vi "Add IP Address.vi"(7 "Connected(F)":bool, 8 "error in":errorcluster, 10 "Alias":string, 11 "IP Address":string) -> (0 "error out":errorcluster, 2 "Alias to Add":string, 3 "IP to Add":string)   [LabVIEW 2014, in "Raspberry Pi Compatible Compiler for LabVIEW.lvlib"]
uses:
  Raspberry Pi Compatible Compiler for LabVIEW.lvlib
  RasPi_Services/Autodetect/Autodetect.lvlib
panel:
  out "Animated Image":i16(ring) caption="Ring 2"
  in  "Cancel":bool
  in  "Add Ip":bool
  in  "Veirfy Connectivity":bool
  in  "Alias":string
  in  "IP Address":string
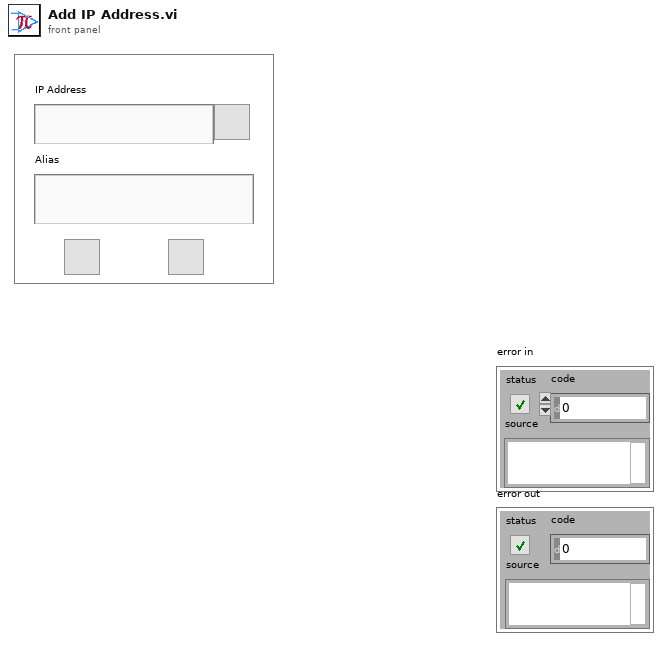
[diagram p1: front panel]
types:
  T1 = enum8{"Enabled", "Disabled", "Disabled and Grayed Out"}
  T2 = typedef "Raspberry Pi Compatible Compiler for LabVIEW.lvlib/Autodetect.lvlib/UDP_Response_TD.ctl" = cluster{"IP address":string, "Port":u16, "response":string}
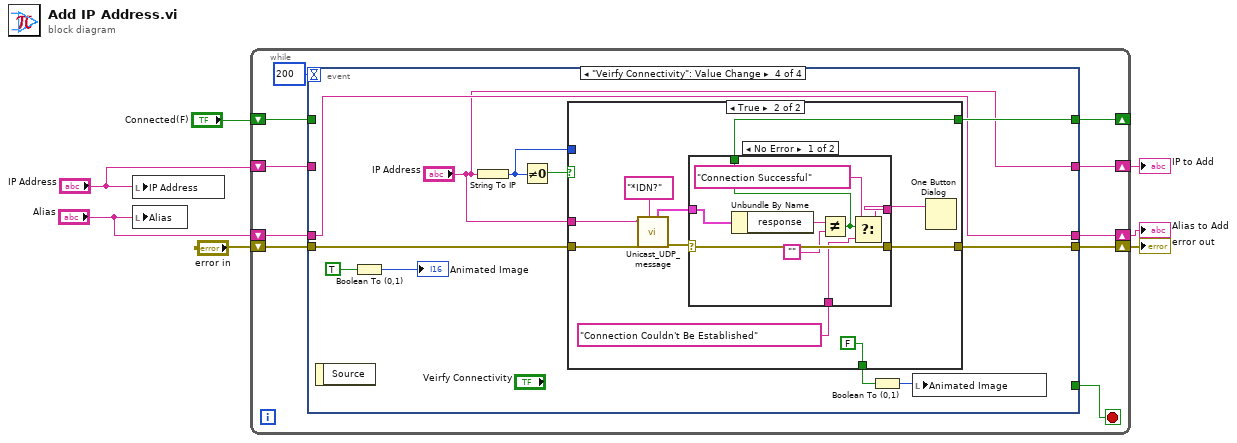
[diagram p0: block diagram]
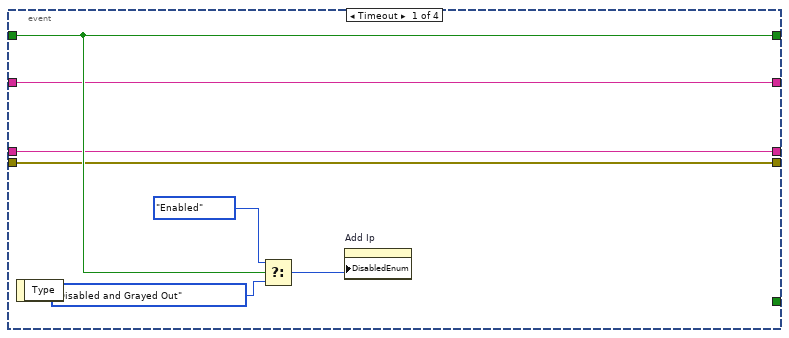
[diagram p2: hidden frame]
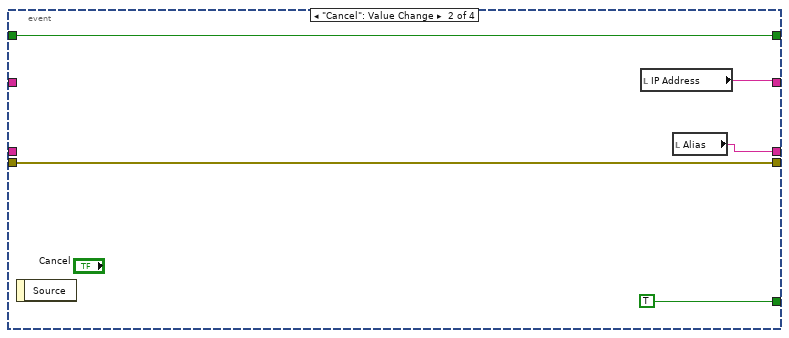
[diagram p3: hidden frame]
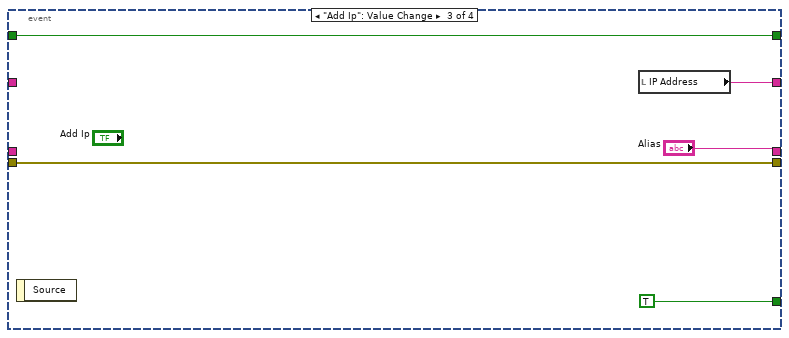
[diagram p4: hidden frame]
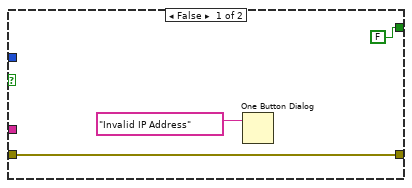
[diagram p5: hidden frame]
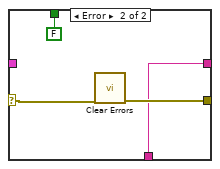
[diagram p6: hidden frame]
diagram:
  n1 = local write "IP Address"("IP Address") -> ()
  n2 = local write "Alias"("Alias") -> ()
  n3 = while {
    shift-right: [w13] -> _
    shift-left: "Connected(F)" -> [w16]
    shift-right: [w14] -> w4
    shift-left: "error in" -> [w15]
    shift-right: [w11] -> w5
    shift-left: "IP Address" -> [w10]
    shift-right: [w9] -> w1
    shift-left: "Alias" -> [w8]
    stop <- w12 stop-if-true
    n4 = event shown="[3] \"Veirfy Connectivity\": Value Change" {
      selector: _ -> [_ _ _ _]
      dyn-events: _ -> [_ _ _ _]
      timeout: 200 -> [_ _ _ _]
      tunnel: w16 -> [w24 w29 w34 _]
      tunnel: w15 -> [w20 w28 w33 w43]
      tunnel: [w20 w28 w33 w42] -> w14
      tunnel: [w24 w29 w34 w41] -> w13
      tunnel: [_ TRUE TRUE _] -> w12
      tunnel: [w19 w26 w30 "IP Address"] -> w11
      tunnel: w10 -> [w19 _ _ _]
      tunnel: [w18 w25 "Alias" w40] -> w9
      tunnel: w8 -> [w18 _ _ w40]
      event Timeout {
        n5 = event-data() -> ()  [unwired: 1 in, 1 out]
        n6 = Select(t=T1."Enabled" ("Disabled"), s=w24, f=T1."Disabled and Grayed Out" ("Disabled")) -> (s? t:f=w22:T1)
        n7 = property on="Add Ip" class="Bool"("DisabledEnum"=w22) -> ()  [unwired: 2 in, 2 out]
      }
      event "Cancel": Value Change {
        n8 = event-data() -> ()  [unwired: 1 in, 1 out]
        n9 = local read "IP Address"() -> (w26:string)
        n10 = local read "Alias"() -> (w25:string)
      }
      event "Add Ip": Value Change {
        n11 = event-data() -> ()  [unwired: 1 in, 1 out]
        n12 = local read "IP Address"() -> (w30:string)
      }
      event "Veirfy Connectivity": Value Change {
        n13 = event-data() -> ()  [unwired: 1 in, 1 out]
        n14 = Boolean To (0,1)(Boolean=TRUE) -> (0, 1=→"Animated Image":i16)
        n15 = String To IP(1:"IP Address") -> (0:w44:u32)
        n16 = Not Equal To 0?(x=w44) -> (x != 0?=w45:bool)
        n17 = case shown="True" w45 {
          tunnel: w44 -> [_ _]
          tunnel: "IP Address" -> [_ w52]
          tunnel: w43 -> [w48 w53]
          tunnel: [w48 w58] -> w42
          tunnel: [FALSE w57] -> w41
          tunnel: [_ FALSE] -> w35
          frame False {
            n18 = One Button Dialog(message="Invalid IP Address") -> ()  [unwired: 1 in, 1 out]
          }
          frame True {
            n19 = call "Unicast_UDP_message.vi"("message"="*IDN?", "error in"=w53, "address"=w52) -> ("error out"=w50:errorcluster, "response"=w49:T2)  [unwired: 5 in]
            n20 = case shown="No Error" w50 {
              selector: w50 -> [w66 w68]
              tunnel: [w66 w70] -> w58
              tunnel: [w62 FALSE] -> w57
              tunnel: [w61 w67] -> w55
              tunnel: "Connection Couldn't Be Established" ("response") -> [w59 w67]
              tunnel: w49 -> [w63 _]
              frame No Error {
                n21 = Unbundle By Name(w63) -> ("response"=w65:string)
                n22 = Not Equal?(x=w65, y="") -> (x != y?=w62:bool)
                n23 = Select(t="Connection Successful" ("response"), s=w62, f=w59) -> (s? t:f=w61:string)
              }
              frame Error {
                n24 = call <vilib>:"Clear Errors.vi"("error in (no error)"=w68) -> ("error out"=w70:errorcluster)  [unwired: 5 in, 1 out]
              }
            }
            n25 = One Button Dialog(message=w55) -> ()  [unwired: 1 in, 1 out]
          }
        }
        n26 = Boolean To (0,1)(Boolean=w35) -> (0, 1=w36:i16)
        n27 = local write "Animated Image"(w36) -> ()
      }
    }
  }
  "IP to Add" <- w5
  "Alias to Add" <- w1
  "error out" <- w4
